vi "Start Calibrate.vi"(0 "CART TCP Connection In":refnum<k5>, 5 "Send Cal Command?":bool=TRUE, 7 "Calibrate Config":T1={"Frequency, MHz"=2412, "TX Gain"=0, "Data Rate"="1,0,0", "Packet Length"=4, "Packet Count"=4}, 9 "Chain Mask":u32=1 format="%x", 11 "error in (no error)":errorcluster) -> (4 "CART TCP Connection Out":refnum<k5>, 6 "Messages Logged":string[](array[string]), 8 "More Pwr Reporting?":bool, 14 "Command Sent":string, 15 "error out":errorcluster)   [LabVIEW 2012]
uses:
  WLAN Reference/WLAN/UUT/QCA/Controls/QCA NART Response Type.ctl
  WLAN Reference/WLAN/UUT/QCA/Controls/QCA NART Response SubType.ctl
  WLAN Reference/WLAN/UUT/QCA/NART Constants.vi
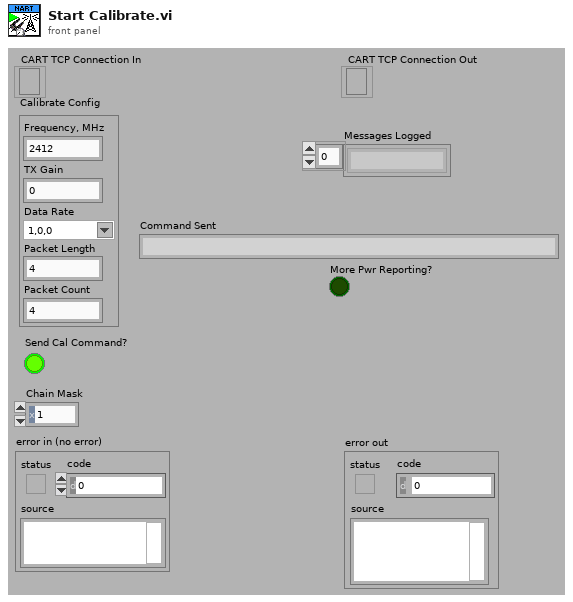
[diagram p1: front panel]
types:
  T1 = cluster{"Frequency, MHz":u32, "TX Gain":u32, "Data Rate":string, "Packet Length":u32, "Packet Count":i32}
  T2 = typedef "QCA NART Response Type.ctl" = enum16{"DEBUG", "CONTROL", "INFO", "WARNING", "ERROR", "NONE"}
  T3 = enum16{"none", "combined", "isolated", "iterate-combined ", "iterate-isolated"}
  T4 = cluster{"Name":string, "Type":enum16{"decimal", "string", "float", "hex"}}[]
  T5 = typedef "QCA NART Response SubType.ctl" = enum16{"NONE", "OK", "ON", "OFF", "BEGIN", "DONE"}
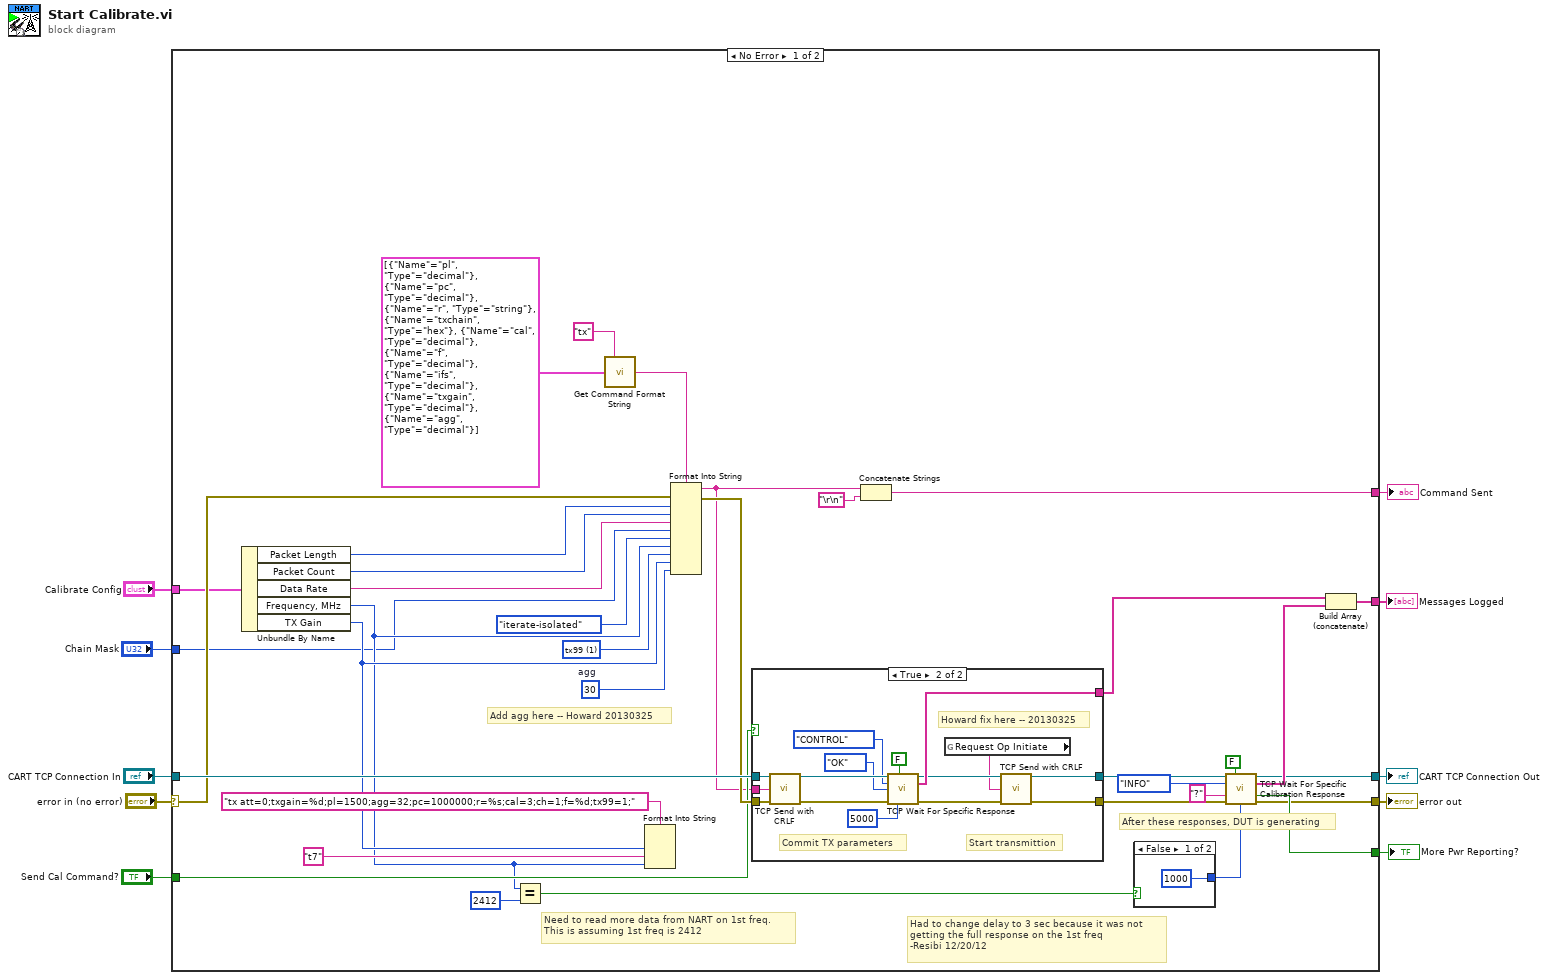
[diagram p0: block diagram]
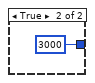
[diagram p2: hidden frame]
diagram:
  n1 = case shown="No Error" "error in (no error)" {
    selector: "error in (no error)" -> [w45 w67]
    tunnel: [w19 w67] -> w9
    tunnel: "CART TCP Connection In" -> [w46 w66]
    tunnel: [w20 w66] -> w7
    tunnel: "Calibrate Config" -> [w43 _]
    tunnel: [w39 _] -> w5
    tunnel: [w32 _] -> w4
    tunnel: [w22 _] -> w3
    tunnel: "Send Cal Command?" -> [w18 _]
    tunnel: "Chain Mask" -> [w11 _]
    frame No Error {
      w13 = u32 30  # agg
      w30 = i16 1 items=["Regular"=-1, "tx100"=0, "tx99"=1] ("Inter Frame Spacing")
      # "Add agg here -- Howard 20130325"
      # "Need to read more data from NART on 1st freq.\nThis is assuming 1st freq is 2412"
      # "Had to change delay to 3 sec because it was not \ngetting the full response on the 1st freq\n-Resibi 12/20/12"
      # "After these responses, DUT is generating"
      n2 = Unbundle By Name(w43) -> ("Packet Length"=w42:u32, "Packet Count"=w36:i32, "Data Rate"=w25:string, "Frequency, MHz"=w16:u32, "TX Gain"=w26:u32)
      n3 = Equal?(x=w16, y=2412) -> (x = y?=w15:bool)
      n4 = call "Get Command Format String.vi"("Command"="tx", "Parameters"=T4 [{"Name"="pl", "Type"=enum."decimal"}, {"Name"="pc", "Type"=enum."decimal"}, {"Name"="r", "Type"=enum."string"}, {"Name"="txchain", "Type"=enum."hex"}, {"Name"="cal", "Type"=enum."decimal"}, {"Name"="f", "Type"=enum."decimal"}, {"Name"="ifs", "Type"=enum."decimal"}, {"Name"="txgain", "Type"=enum."decimal"}, {"Name"="agg", "Type"=enum."decimal"}]) -> ("Command Format String"=w33:string)  [unwired: 13 in]
      n5 = Format Into String(format string="tx att=0;txgain=%d;pl=1500;agg=32;pc=1000000;r=%s;cal=3;ch=1;f=%d;tx99=1;" ("Name"), w26, "t7" ("input 2"), w16) -> ()  [unwired: 2 in, 2 out]
      n6 = Format Into String(format string=w33, error in=w45, w42, w36, w25, w11, T3."iterate-isolated" ("Calibrate TXP"), w16, w30, w26, w13) -> (resulting string=w14:string, error out=w44:errorcluster)  [unwired: 1 in]
      n7 = case shown="True" w18 {
        tunnel: w46 -> [w49 w65]
        tunnel: w44 -> [w50 w64]
        tunnel: [_ w62] -> w41
        tunnel: [w49 w57] -> w38
        tunnel: [w50 w56] -> w37
        tunnel: w14 -> [_ w53]
        frame False {
        }
        frame True {
          # "Howard fix here -- 20130325"
          # "Start transmittion"
          # "Commit TX parameters"
          n8 = call "TCP Send with CRLF.vi"("CART TCP Connection"=w65, "data in"=w53, "error IO"=w64) -> ("CART TCP Connection Out"=w61:refnum<k5>, "error out"=w60:errorcluster)  [unwired: 11 in]
          n9 = call "TCP Wait For Specific Response.vi"("TCP Connection In"=w61, "Next response (t)"=FALSE, "Expected Type"=QCA_NART_Response_Type."CONTROL", "Expected Subtype (none)"=QCA_NART_Response_SubType."OK", "error in"=w60, "Timeout (250 ms)"=5000 ("Timeout (100ms)")) -> ("TCP Connection Out"=w58:refnum<k5>, "TCP Messages"=w62:string[], "error out"=w59:errorcluster)  [unwired: 6 in, 1 out]
          n10 = global read "NART Constants.vi" "Request Op Initiate"() -> (w54:string)
          n11 = call "TCP Send with CRLF.vi"("CART TCP Connection"=w58, "data in"=w54, "error IO"=w59) -> ("CART TCP Connection Out"=w57:refnum<k5>, "error out"=w56:errorcluster)  [unwired: 11 in]
        }
      }
      n12 = Concatenate Strings(w14, "\r\n") -> (w32:string)
      n13 = case shown="False" w15 {
        tunnel: [1000 ("Timeout (250 ms)") 3000 ("Timeout (250 ms)")] -> w23
        frame False {
        }
        frame True {
        }
      }
      n14 = call "TCP Wait For Specific Calibration Response.vi"("TCP Connection In"=w38, "Next response (t)"=FALSE, "Expected Type"=QCA_NART_Response_Type."INFO", "Expected Message Start (\"\":any)"="?" ("Expected Message Start (\"\":any)"), "error in"=w37, "Timeout (250 ms)"=w23) -> ("TCP Connection Out"=w20:refnum<k5>, "TCP Messages"=w40:string[], "More Pwr Reporting?"=w22:bool, "error out"=w19:errorcluster)  [unwired: 5 in, 1 out]
      n15 = Build Array (concatenate)(w41, w40) -> (w39:string[])
    }
    frame Error {
    }
  }
  "error out" <- w9
  "CART TCP Connection Out" <- w7
  "Messages Logged" <- w5
  "Command Sent" <- w4
  "More Pwr Reporting?" <- w3
